vi "eFinance.vi"() -> ()   [LabVIEW 2023]
panel:
  out "Line Size":dbl[](array[numeric]) format="%#_1g"
  out "Array 2":string[](array[string])
  out "Array":string[][](array[string])
  out "result string":string
  out "match substring":string
  in  "RowNum":dbl format="%#_2g"
  out "eCents":string
  out "eLev":string
  out "Account":string
  out "Date":string
  out "Table Control":string[][](table)
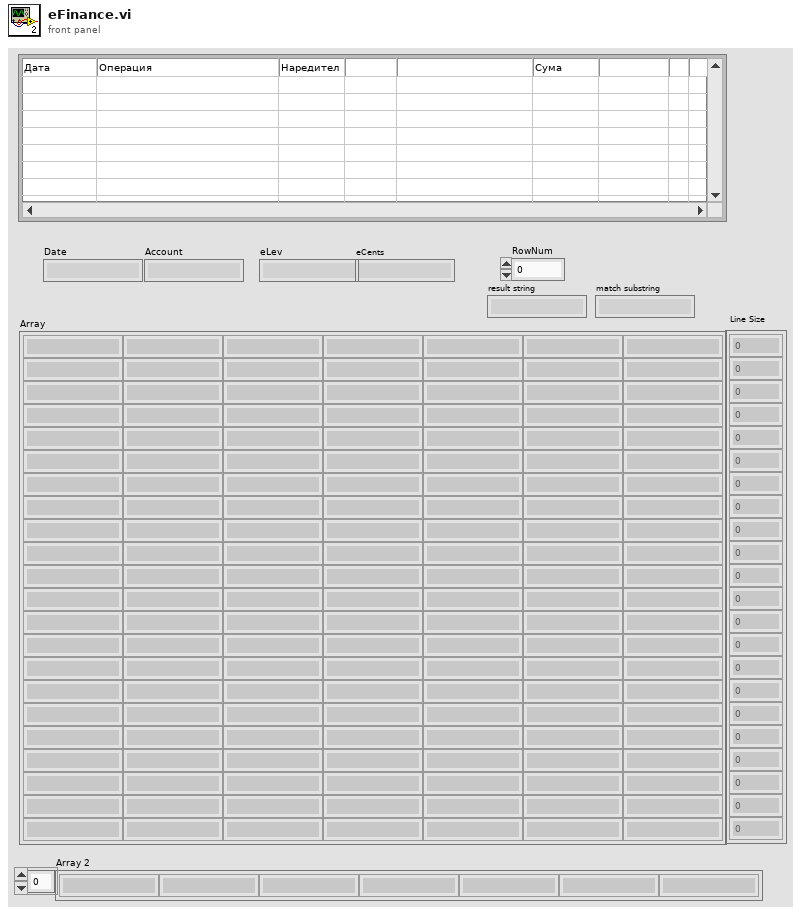
[diagram p1: front panel]
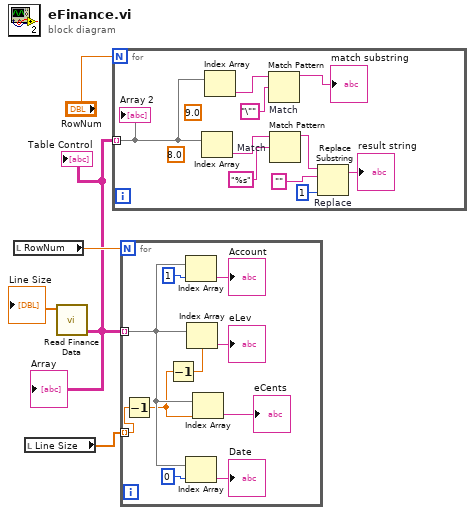
[diagram p0: block diagram]
diagram:
  n1 = local read "RowNum"() -> (w4:dbl)
  n2 = local read "Line Size"() -> (w1:dbl[])
  n3 = call "Read Finance Data.vi"() -> ("Result Array"=w3:string[][], "Line Size"=→"Line Size":dbl[])  [unwired: 10 in]
  "Table Control" <- w3
  "Array" <- w3
  n4 = for {
    N: "RowNum" -> [_]
    tunnel: w3 -> [w6] mode=indexing
    (unwired) 9.0 ("ColNum")
    (unwired) 8.0 ("ColNum")
    n5 = Index Array(array=w6) -> (element=w15:string)  [unwired: 1 in]
    n6 = Index Array(array=w6) -> (element=w13:string)  [unwired: 1 in]
    n7 = Match Pattern "Match"(string=w13, regular expression="\"") -> (before substring=→"match substring":string)  [unwired: 1 in, 3 out]
    n8 = Match Pattern "Match"(string=w15, regular expression="%s") -> (before substring=w8:string)  [unwired: 1 in, 3 out]
    n9 = Replace Substring "Replace"(2:1 ("length (len. of substring)"), 4:"" ("substring (\"\")"), 5:w8) -> (1:→"result string":string)  [unwired: 1 in, 1 out]
    "Array 2" <- w6
  }
  n10 = for {
    N: w4 -> [_]
    tunnel: w3 -> [w19] mode=indexing
    tunnel: w1 -> [w18] mode=indexing
    n11 = Decrement(x=w18) -> (x-1=w17:dbl)
    n12 = Decrement(x=w17) -> (x-1=w16:dbl)
    n13 = Index Array(array=w19, index=1) -> (element=→"Account":string)
    n14 = Index Array(array=w19, index=0) -> (element=→"Date":string)
    n15 = Index Array(array=w19, index=w16) -> (element=→"eLev":string)
    n16 = Index Array(array=w19, index=w17) -> (element=→"eCents":string)
  }
